vi "Register PVs.vi"(8 "error in (no error)":errorcluster, 10 "Activate?":bool, 11 "CS++PVProxy in":refnum<class "CS++PVProxy.lvclass">) -> (0 "error out":errorcluster, 3 "CS++PVProxy out":refnum<class "CS++PVProxy.lvclass">)   [LabVIEW 2015, in "CS++PVProxy.lvlib" / "CS++PVProxy.lvclass"]
uses:
  CS++PVProxy.lvclass
  CS++PVProxy.lvclass/CS++PVProxy.ctl
  CS++PVMonitor Messages/Register PVs Msg/Register PVs Msg.lvclass/Register PVs Msg.ctl
  <vilib>/ActorFramework/Message Enqueuer/Message Enqueuer.lvclass/Message Enqueuer.ctl
  <vilib>/ActorFramework/Message Enqueuer/Enqueue.vi
  <vilib>/ActorFramework/Message Priority Queue/Priority Enqueue.vi
  <vilib>/ActorFramework/Message Enqueuer/Message Enqueuer.lvclass
  CS++PVMonitor Messages/CS++PVUpdate Msg/CS++PVUpdate Msg.lvclass
  CS++PVMonitor Messages/Register PVs Msg/Register PVs Msg.lvclass
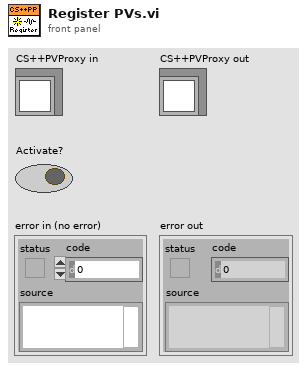
[diagram p1: front panel]
types:
  T1 = cluster{"Accessors:Device Actor's Enqueuer":refnum<class "Message Enqueuer.lvclass">, "Msgs":refnum<class "CS++PVUpdate Msg.lvclass">[]}[]
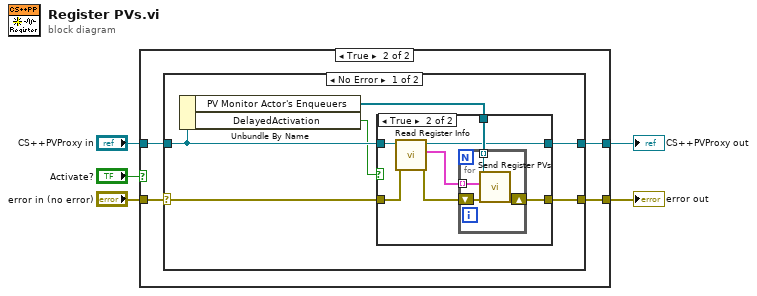
[diagram p0: block diagram]
diagram:
  n1 = case shown="True" "Activate?" {
    tunnel: "error in (no error)" -> [w6 w11]
    tunnel: [w6 w10] -> w4
    tunnel: "CS++PVProxy in" -> [w7 w9]
    tunnel: [w7 w8] -> w2
    frame False {
    }
    frame True {
      n2 = case shown="No Error" w11 {
        selector: w11 -> [w14 w32]
        tunnel: [w13 w32] -> w10
        tunnel: [w15 w31] -> w8
        tunnel: w9 -> [w16 w31]
        frame No Error {
          n3 = Unbundle By Name(w16) -> ("PV Monitor Actor's Enqueuers"=w17:refnum<class "Message Enqueuer.lvclass">[], "DelayedActivation"=w12:bool)
          n4 = case shown="True" w12 {
            tunnel: w17 -> [_ w26]
            tunnel: w16 -> [w19 w25]
            tunnel: [w19 w24] -> w15
            tunnel: w14 -> [w18 w21]
            tunnel: [w18 w20] -> w13
            frame False {
            }
            frame True {
              n5 = call "Read Register Info.vi"("error in (no error)"=w21, "CS++PVProxy in"=w25) -> ("error out"=w22:errorcluster, "Register Info"=w23:T1, "CS++PVProxy out"=w24:refnum<class "CS++PVProxy.lvclass">)  [unwired: 7 in]
              n6 = for {
                tunnel: w26 -> [w30] mode=indexing
                tunnel: w23 -> [w29] mode=indexing
                shift-right: [w27] -> w20
                shift-left: w22 -> [w28]
                n7 = call "Send Register PVs.vi"("error in (no error)"=w28, "Register Info"=w29, "Message Enqueuer"=w30) -> ("error out"=w27:errorcluster)  [unwired: 7 in, 1 out]
              }
            }
          }
        }
        frame Error {
        }
      }
    }
  }
  "error out" <- w4
  "CS++PVProxy out" <- w2
